vi "Log.vi"(8 "error in (no error)":errorcluster, 10 "LogRecord":refnum<class "LogRecord.lvclass">, 11 "LoggingHandle in":refnum<class "LoggingHandle.lvclass">) -> (0 "error out":errorcluster, 3 "LoggingHandle out":refnum<class "LoggingHandle.lvclass">)   [LabVIEW 2024, in "LoggingHandle.lvclass"]
uses:
  LoggingHandle.lvclass
  Record/LogRecord.lvclass
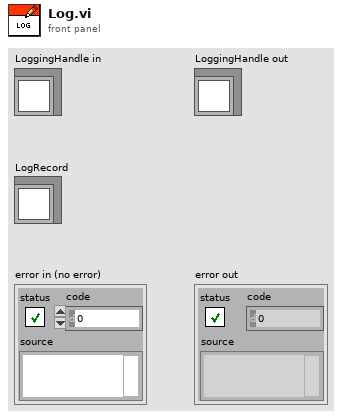
[diagram p1: front panel]
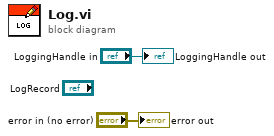
[diagram p0: block diagram]
diagram:
  "error out" <- "error in (no error)"
  "LoggingHandle out" <- "LoggingHandle in"
